vi "turning with gyro (1).vi"(7 "desired angle":dbl=45.0 format="%#_13g", 8 "error in (no error)":errorcluster, 11 "RobotDriveDevRef":T1={"DevStatus"={"status"=FALSE, "code"=0, "source"=""}, "Motors[]"=[], "Square Inputs"=FALSE, "Max Output"=1.0}) -> (0 "error out":errorcluster, 3 "RobotDriveDevRef 2":T1={"DevStatus"={"status"=FALSE, "code"=0, "source"=""}, "Motors[]"=[], "Square Inputs"=FALSE, "Max Output"=1.0})   [LabVIEW 2016]
uses:
  <vilib>/Rock Robotics/WPI/RobotDrive/WPI_RobotDriveDevRef.ctl
  <vilib>/Rock Robotics/WPI/MotorControl/WPI_MotorControlDeviceRef.ctl
  <vilib>/Rock Robotics/WPI/MotorControl/WPI_MotorControlType.ctl
  <vilib>/Rock Robotics/SystemInterfaces/DIO/FPGA_DIOPWMChannel.ctl
  <vilib>/Rock Robotics/WPI/PWM/WPI_PWMDeadband.ctl
  <vilib>/Rock Robotics/WPI/RobotDrive/WPI_RobotDriveArcadeDrive_Standard(NoSaturation).vi
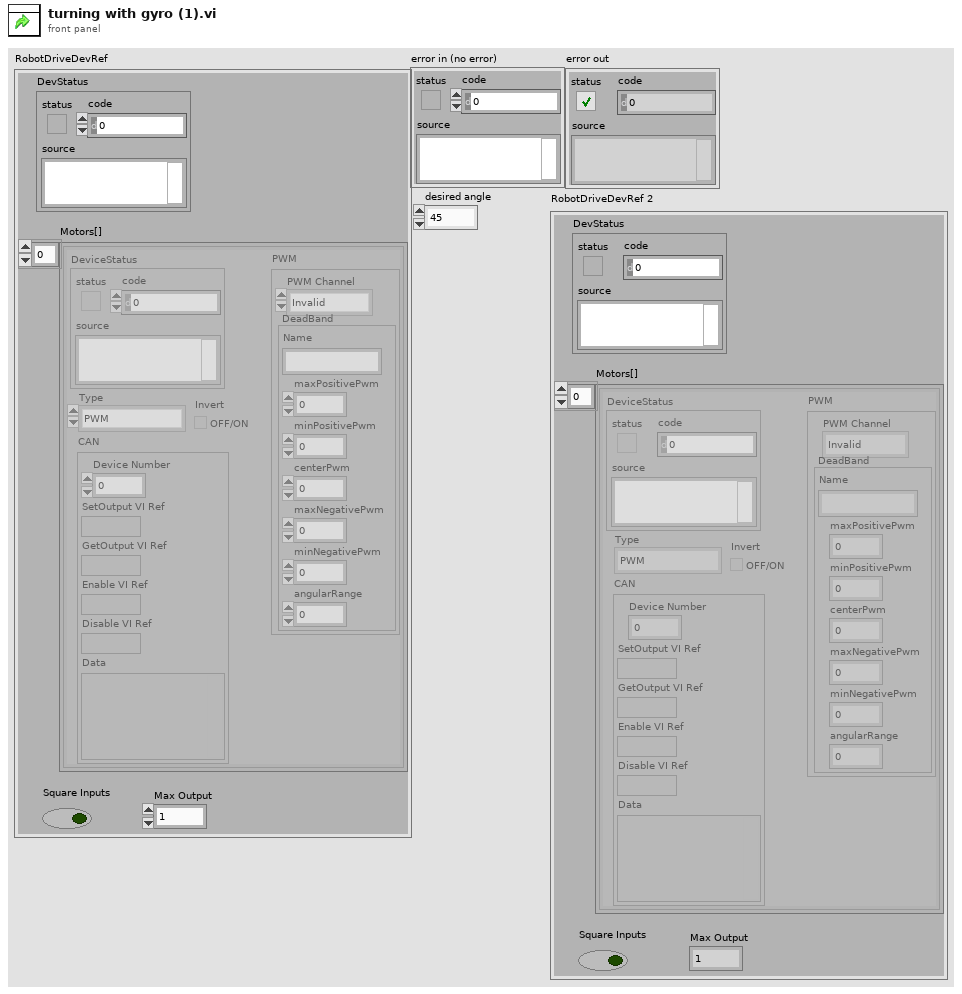
[diagram p1: front panel]
types:
  T1 = typedef "WPI_RobotDriveDevRef.ctl" = cluster{"DevStatus":errorcluster, "Motors[]":T2[], "Square Inputs":bool, "Max Output":dbl}
  T2 = typedef "WPI_MotorControlDeviceRef.ctl" = cluster{"DeviceStatus":errorcluster, "Type":T3, "PWM":cluster{"PWM Channel":T4, "DeadBand":T5}, "CAN":cluster{"Device Number":u8, "SetOutput VI Ref":variant, "GetOutput VI Ref":variant, "Enable VI Ref":variant, "Disable VI Ref":variant, "Data":variant}, "Invert":bool}
  T3 = typedef "WPI_MotorControlType.ctl" = enum16{"PWM", "CAN"}
  T4 = typedef "FPGA_DIOPWMChannel.ctl" = enum8{"PWM 0", "PWM 1", "PWM 2", "PWM 3", "PWM 4", "PWM 5", "PWM 6", "PWM 7", "PWM 8", "PWM 9", "PWM MXP 0", "PWM MXP 1", "PWM MXP 2", "PWM MXP 3", "PWM MXP 4", "PWM MXP 5", "PWM MXP 6", "PWM MXP 7", "PWM MXP 8", "PWM MXP 9", "Invalid"}
  T5 = typedef "WPI_PWMDeadband.ctl" = cluster{"Name":string, "maxPositivePwm":i32, "minPositivePwm":i32, "centerPwm":i32, "maxNegativePwm":i32, "minNegativePwm":i32, "angularRange":u16}
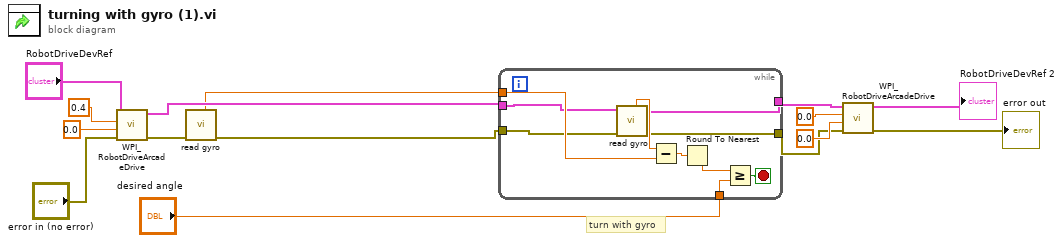
[diagram p0: block diagram]
diagram:
  # "turn with gyro"
  n1 = call-poly <vilib>:"WPI_RobotDriveArcadeDrive.vi"("error in (no error)"="error in (no error)", "Y axis value"=0.0 ("X axis value"), "X axis value"=0.4, "RobotDriveDevRef"="RobotDriveDevRef") -> ("error out"=w13:errorcluster, "RobotDriveDevRef"=w11:T1)  [unwired: 6 out]
  n2 = call "read gyro.vi"("error in (no error)"=w13) -> ("error out"=w12:errorcluster, "Angle 2"=w10:dbl)  [unwired: 9 in]
  n3 = while {
    tunnel: w12 -> [w16]
    tunnel: w11 -> [w17]
    tunnel: w10 -> [w23]
    tunnel: [w20] -> w7
    tunnel: [w17] -> w6
    tunnel: "desired angle" -> [w19]
    stop <- w21 stop-if-true
    n4 = call "read gyro.vi"("error in (no error)"=w16) -> ("error out"=w20:errorcluster, "Angle 2"=w24:dbl)  [unwired: 9 in]
    n5 = Subtract(x=w24, y=w23) -> (x-y=w18:dbl)
    n6 = Round To Nearest(number=w18) -> (nearest integer value=w22:dbl)
    n7 = Greater Or Equal?(x=w22, y=w19) -> (x >= y?=w21:bool)
  }
  n8 = call-poly <vilib>:"WPI_RobotDriveArcadeDrive.vi"("error in (no error)"=w7, "Y axis value"=0.0, "X axis value"=0.0, "RobotDriveDevRef"=w6) -> ("error out"=→"error out":errorcluster, "RobotDriveDevRef"=→"RobotDriveDevRef 2":T1)  [unwired: 6 out]
